vi "SOURCE_CURR_B2900.vi"() -> ()   [LabVIEW 2020]
panel:
  out "output string":string
  in  "Source Range Lower Limit (2 V)":dbl=2.0
  in  "Source Auto Range (T: Enable)":bool=TRUE
  in  "Channel (0: Channel 1)":i32(ring) items=["Channel 1", "Channel 2"]
  in  "Enable Continuous Output (T: Enable)":bool=TRUE
  in  "Source Range (2)":dbl=2.0
  in  "Source Shape (1: DC)":i32(ring)=1 items=["Pulse", "DC"]
  in  "Source Mode (1: Voltage)":i32(ring)=1 items=["Current", "Voltage"]
  in  "Triggered Output Level (0)":dbl
  in  "Output Level (0)":dbl
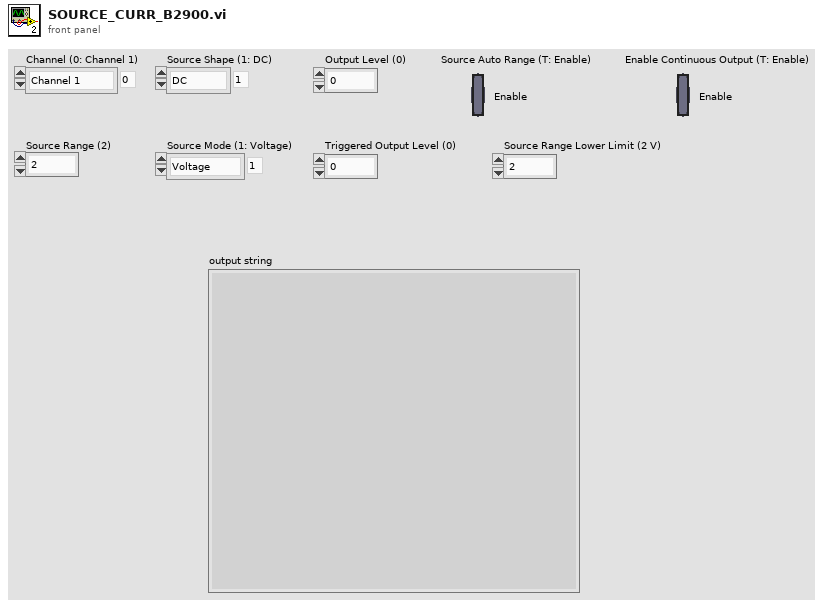
[diagram p1: front panel]
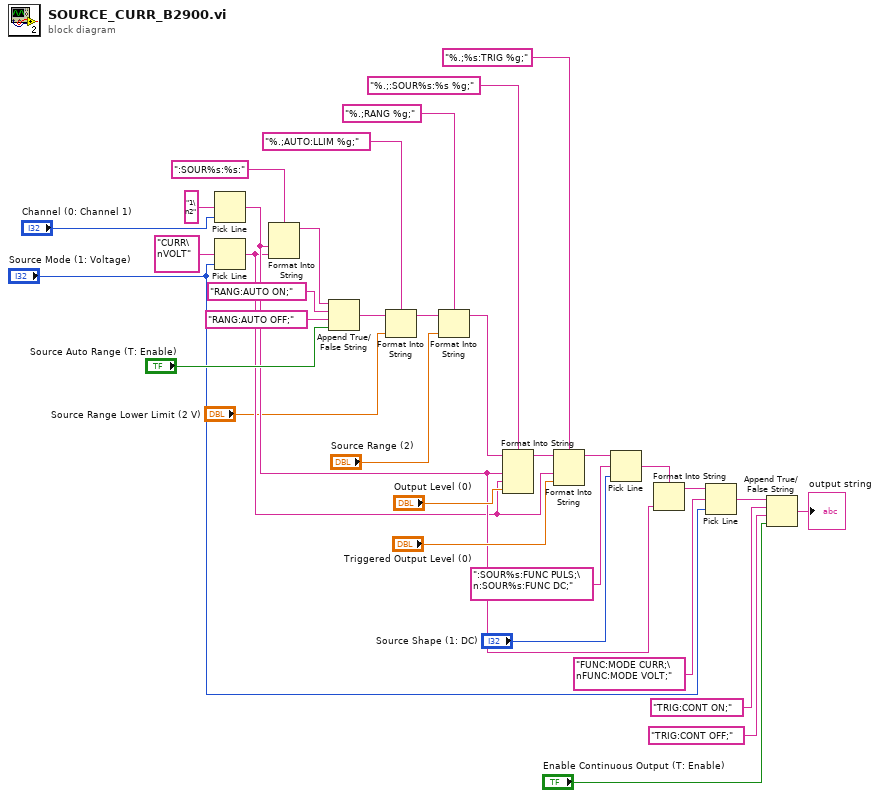
[diagram p0: block diagram]
diagram:
  n1 = Pick Line(multi-line string="1\n2" ("string (\"\")"), line index="Channel (0: Channel 1)") -> (output string=w9:string)  [unwired: 1 in]
  n2 = Pick Line(multi-line string="CURR\nVOLT" ("string (\"\")"), line index="Source Mode (1: Voltage)") -> (output string=w8:string)  [unwired: 1 in]
  n3 = Format Into String(format string=":SOUR%s:%s:", w9, w8) -> (resulting string=w6:string)  [unwired: 2 in, 1 out]
  n4 = Append True/False String(1:"Source Auto Range (T: Enable)", 2:"RANG:AUTO OFF;", 3:"RANG:AUTO ON;", 4:w6) -> (0:w3:string)
  n5 = Format Into String(format string="%.;AUTO:LLIM %g;", initial string=w3, "Source Range Lower Limit (2 V)") -> (resulting string=w5:string)  [unwired: 1 in, 1 out]
  n6 = Format Into String(format string="%.;RANG %g;", initial string=w5, "Source Range (2)") -> (resulting string=w15:string)  [unwired: 1 in, 1 out]
  n7 = Format Into String(format string="%.;:SOUR%s:%s %g;", initial string=w15, w9, w8, "Output Level (0)") -> (resulting string=w32:string)  [unwired: 1 in, 1 out]
  n8 = Format Into String(format string="%.;%s:TRIG %g;", initial string=w32, w8, "Triggered Output Level (0)") -> (resulting string=w14:string)  [unwired: 1 in, 1 out]
  n9 = Pick Line(string ("")=w14, multi-line string=":SOUR%s:FUNC PULS;\n:SOUR%s:FUNC DC;", line index="Source Shape (1: DC)") -> (output string=w22:string)
  n10 = Format Into String(format string=w22, w9) -> (resulting string=w21:string)  [unwired: 2 in, 1 out]
  n11 = Pick Line(string ("")=w21, multi-line string="FUNC:MODE CURR;\nFUNC:MODE VOLT;", line index="Source Mode (1: Voltage)") -> (output string=w20:string)
  n12 = Append True/False String(1:"Enable Continuous Output (T: Enable)", 2:"TRIG:CONT OFF;", 3:"TRIG:CONT ON;", 4:w20) -> (0:→"output string":string)
